vi "Solve1.vi"(8 "Error In":errorcluster, 11 "object in":refnum<class "2022_7.lvclass">) -> (0 "Error Out":errorcluster, 2 "Result":u64, 3 "object out":refnum<class "2022_7.lvclass">)   [LabVIEW 2020, in "2022_7.lvclass"]
uses:
  2022_7.lvclass
  2022_7.lvclass/2022_7.ctl
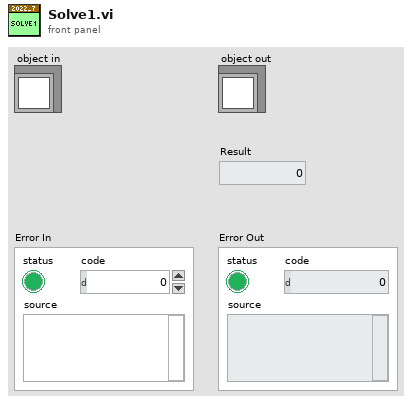
[diagram p1: front panel]
types:
  T1 = map{string[], cluster{"Folders":string[], "Files":cluster{"Name":string, "Size":i32}[]}}
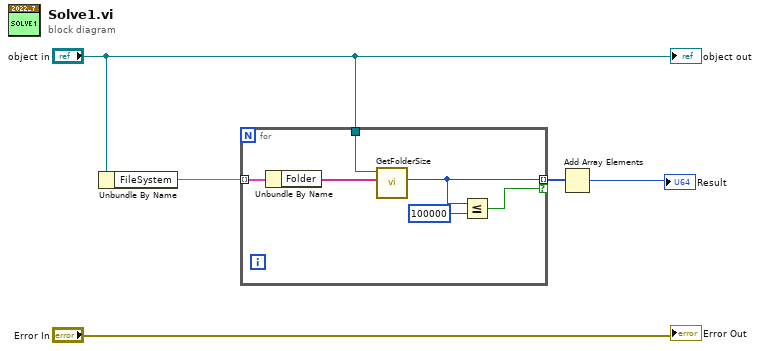
[diagram p0: block diagram]
diagram:
  n1 = Unbundle By Name("object in") -> ("FileSystem"=w4:T1)
  n2 = for {
    tunnel: w4 -> [w11] mode=indexing
    tunnel: "object in" -> [w9]
    tunnel: [w8] -> w2 mode=indexing if=w6
    n3 = Unbundle By Name(w11) -> ("Folder"=w10:string[])
    n4 = call "GetFolderSize.vi"("Folder"=w10, "object in"=w9) -> ("Size"=w8:u64)  [unwired: 7 in, 2 out]
    n5 = Less Or Equal?(x=w8, y=u64 100000) -> (x <= y?=w6:bool)
  }
  n6 = Add Array Elements(numeric array=w2) -> (sum=→"Result":u64)
  "Error Out" <- "Error In"
  "object out" <- "object in"
